vi "LVClass_ClosedLoopSecurity Read ClosedLoopSecurity.vi"(8 "error in (no error)":errorcluster, 11 "ClosedLoopSecurity in":refnum<class "ClosedLoopSecurity.lvclass">) -> (0 "error out":errorcluster, 2 "ClassID_void":T1, 3 "ClosedLoopSecurity out":refnum<class "ClosedLoopSecurity.lvclass">)   [LabVIEW 2020, in "ClosedLoopSecurity.lvclass"]
uses:
  ClosedLoopSecurity.lvclass
  ClassID.ctl
  ClosedLoopSecurity.lvclass/ClosedLoopSecurity.ctl
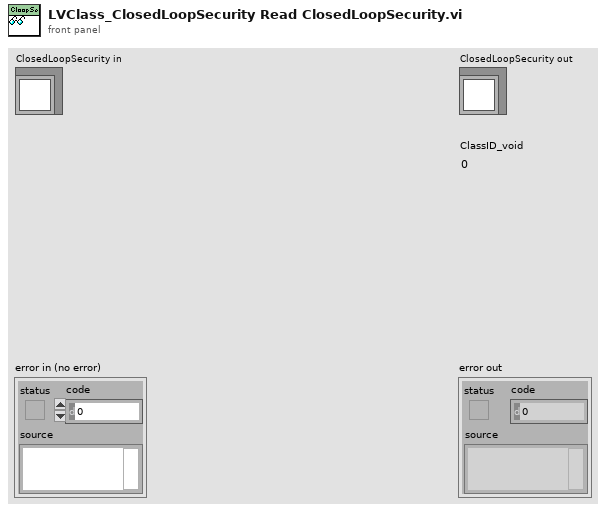
[diagram p1: front panel]
types:
  T1 = typedef "ClassID.ctl" = i64
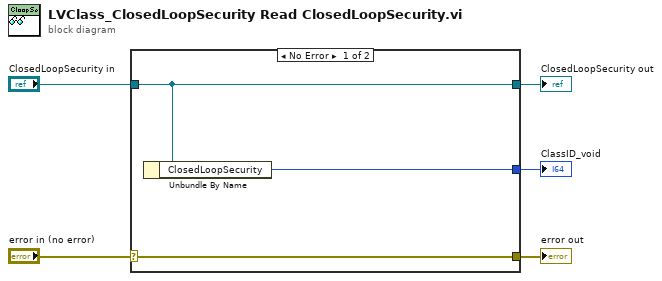
[diagram p0: block diagram]
diagram:
  n1 = case shown="No Error" "error in (no error)" {
    selector: "error in (no error)" -> [w8 w9]
    tunnel: [w8 w9] -> w4
    tunnel: [w7 w10] -> w2
    tunnel: "ClosedLoopSecurity in" -> [w7 w10]
    tunnel: [w6 _] -> w1
    frame No Error {
      n2 = Unbundle By Name(w7) -> ("ClosedLoopSecurity"=w6:T1)
    }
    frame Error {
    }
  }
  "error out" <- w4
  "ClosedLoopSecurity out" <- w2
  "ClassID_void" <- w1
